vi "FTW-Actor-Destroy.vi"(0 "FTW Actor Instance":refnum<class "FTW-Actor-Instance.lvclass">, 11 "error in":errorcluster) -> (15 "error out":errorcluster)   [LabVIEW 2014, in "FTW-Actor-Instance.lvclass"]
uses:
  FTW-Actor-Instance.lvclass
  FTW-Actor-Instance.lvclass/FTW-Actor-Instance.ctl
  logger/FTW-Logger.lvclass
  scheduler/FTW-Scheduler.lvclass
  router/FTW-Router.lvclass
panel:
  # "Inputs"
  # "Outputs"
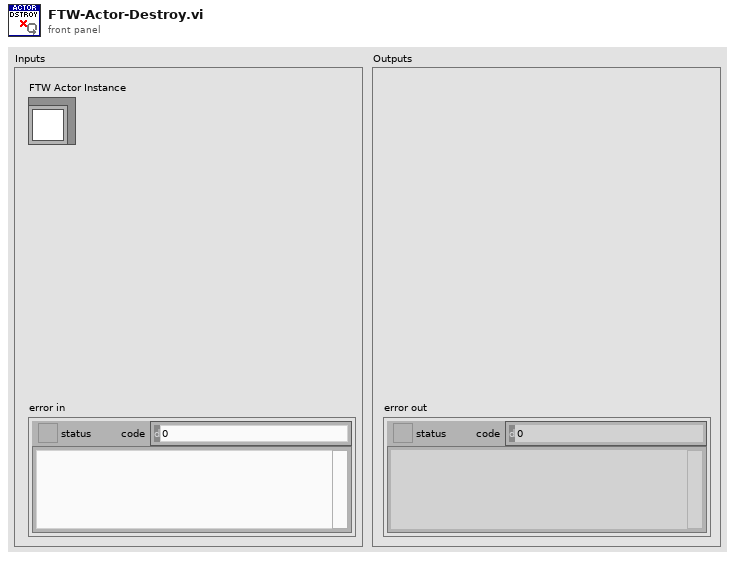
[diagram p1: front panel]
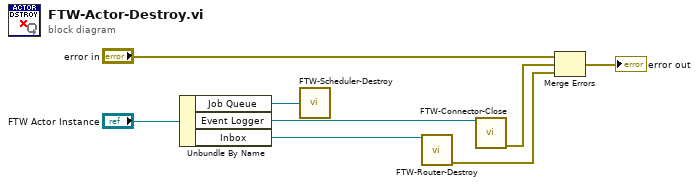
[diagram p0: block diagram]
diagram:
  n1 = Unbundle By Name("FTW Actor Instance") -> ("Job Queue"=w5:refnum<class "FTW-Scheduler.lvclass">, "Event Logger"=w2:refnum<class "FTW-Logger.lvclass">, "Inbox"=w3:refnum<class "FTW-Router.lvclass">)
  n2 = call "FTW-Scheduler-Destroy.vi"("FTW Job Scheduler"=w5) -> ()  [unwired: 1 in]
  n3 = call "FTW-Router-Destroy.vi"("FTW Router"=w3) -> ("error out"=w4:errorcluster)  [unwired: 14 in]
  n4 = call-dynamic "FTW-Connector-Close.vi"("FTW Actor Connector"=w2) -> ("error out"=w1:errorcluster)  [unwired: 14 in]
  n5 = Merge Errors("error in", w1, w4) -> (→"error out":errorcluster)
